vi "comms_Serial_Send_Com.vi"(8 "error in":errorcluster, 9 "Buffer Clear?":bool, 10 "Command":string, 11 "VISA resource in":refnum<visa-resource-name>) -> (0 "error out":errorcluster, 2 "Response":string, 3 "VISA resource Out":refnum<visa-resource-name>)   [LabVIEW 2018]
panel:
  out "return count":u32
  out "cleared data":string
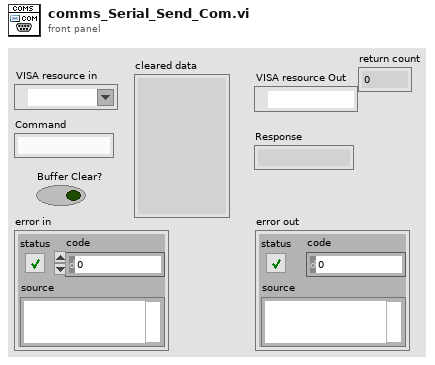
[diagram p1: front panel]
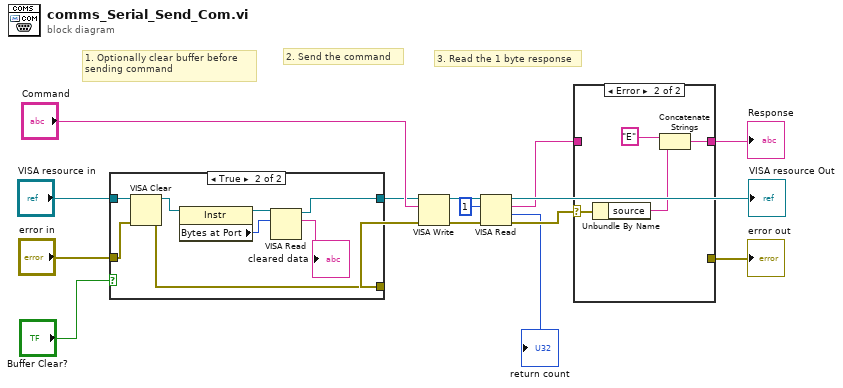
[diagram p0: block diagram]
diagram:
  # "3. Read the 1 byte response"
  # "2. Send the command"
  # "1. Optionally clear buffer before \nsending command"
  n1 = case shown="True" "Buffer Clear?" {
    tunnel: "VISA resource in" -> [w17 w25]
    tunnel: [w17 w19] -> w7
    tunnel: "error in" -> [w16 w24]
    tunnel: [w16 w23] -> w10
    frame False {
    }
    frame True {
      n2 = VISA Clear(VISA resource name=w25, error in (no error)=w24) -> (VISA resource name out=w20:refnum<visa-resource-name>, error out=w23:errorcluster)
      n3 = property class="Instr"(reference=w20) -> (reference out=w21:refnum<visa-resource-name>, "Bytes at Port"=w22:u32)  [unwired: 1 in, 1 out]
      n4 = VISA Read(VISA resource name=w21, byte count=w22) -> (VISA resource name out=w19:refnum<visa-resource-name>, read buffer=→"cleared data":string)  [unwired: 1 in, 2 out]
    }
  }
  n5 = VISA Write(VISA resource name=w7, write buffer="Command", error in (no error)=w10) -> (VISA resource name out=w6:refnum<visa-resource-name>, error out=w9:errorcluster)  [unwired: 1 out]
  n6 = VISA Read(VISA resource name=w6, byte count=u32 1, error in (no error)=w9) -> (VISA resource name out=→"VISA resource Out":refnum<visa-resource-name>, read buffer=w3:string, return count=→"return count":u32, error out=w5:errorcluster)
  n7 = case shown="Error" w5 {
    selector: w5 -> [w27 w31]
    tunnel: [w27 _] -> w4
    tunnel: w3 -> [w26 _]
    tunnel: [w26 w30] -> w2
    frame No Error {
    }
    frame Error {
      n8 = Unbundle By Name(w31) -> ("source"=w29:string)
      n9 = Concatenate Strings("E", w29) -> (w30:string)
    }
  }
  "error out" <- w4
  "Response" <- w2
